vi "Esophogeal_HRME_Main_ImageCasting.vi"() -> ()   [LabVIEW 2021]
uses:
  typeDefs/Esophogeal_Software_States.ctl
  <vilib>/Utility/miscctls.llb/LVAllMonitorsDisplayTypeDef.ctl
  <vilib>/DAQmx/read.llb/DAQmx Read (Digital 1D Bool NChan 1Samp 1Line).vi
  <extravilib>/ChannelInstances/High Speed Stream-str/_Read For Replicate.vi
  <extravilib>/ChannelInstances/High Speed Stream-a[.,.](u8)/_Read For Replicate.vi
  <vilib>/DAQmx/create/channels.llb/DAQmx Create Channel (DI-Digital Input).vi
  <vilib>/DAQmx/miscellaneous.llb/DAQmx Fill In Error Info.vi
  <extravilib>/ChannelInstances/High Speed Stream-str/Instantiate.vi
  <extravilib>/ChannelInstances/High Speed Stream-a[.,.](u8)/Instantiate.vi
  <extravilib>/ChannelInstances/High Speed Stream-str/)Channel.vi
  <extravilib>/ChannelInstances/High Speed Stream-str/Abort Signal/Init Signal.vi
  <extravilib>/ChannelInstances/High Speed Stream-a[.,.](u8)/)Channel.vi
  <extravilib>/ChannelInstances/High Speed Stream-a[.,.](u8)/Abort Signal/Init Signal.vi
  <vilib>/vision/driver/NI_Vision_Acquisition_Software.lvlib
  <resource>/objmgr/imaqdx.rc
  <extravilib>/ChannelInstances/High Speed Stream-a[.,.](u8).lvlib
  <extravilib>/ChannelInstances/High Speed Stream-str.lvlib
  <vilib>/vision/NI_Vision_Development_Module.lvlib
panel:
  out "Pause Status":bool
  in  "Tab Control":enum32{"Main Page", "Image Session Info"}(tab)
  in  "MTN Threshold:":enum16{"24.0", "15.9"}(ring)
  in  "Calibrate":bool
  out "Image Analysis Meter":dbl(slide) scale=0.0..100.0
  out "Saved Imaged Number":i32=1 caption="Number of Images Saved"
  out "Image Save Notification":string
  in  "Auto Gain":bool=TRUE
  in  "Auto Exposure":bool=TRUE
  in  "Save Button":bool
  out "Recording":bool
  in  "Play Button":bool
  in  "Pause Button":bool
  in  "Close Program":bool
  in  "HRME Gain":dbl(slide)=18.0 scale=0.0..30.0
  in  "HRME Exposure":dbl(slide)=7000.0 scale=100.0..80000.0
  out "HRME Image":T1(plugin-control)
  out "Software States":T2
  out "HRME Path":path
  out "HRME Scores":path
  out "Representative Images":path
  out "error out":errorcluster
  out "Patient Folder":path
  in  "Command File Location":path=path "C:/Users/EsophaHRME_Dell3/Documents/GitHub/Esophageal_HRME_Software/EsophagealDeployment/Multi_Task_Network/CommandFiles/LabVIEW/cmds.json"
  out "Display:All Monitors":T3
  out "Width":i16
  out "Height":i16
  in  "Python Module Path":path=path "C:/Users/EsophaHRME_Dell3/Documents/GitHub/Esophageal_HRME_Software/EsophagealDeployment/Multi_Task_Network/mainv6.py"
  out "Log File Out":refnum<file>
  out "Timestamp":string
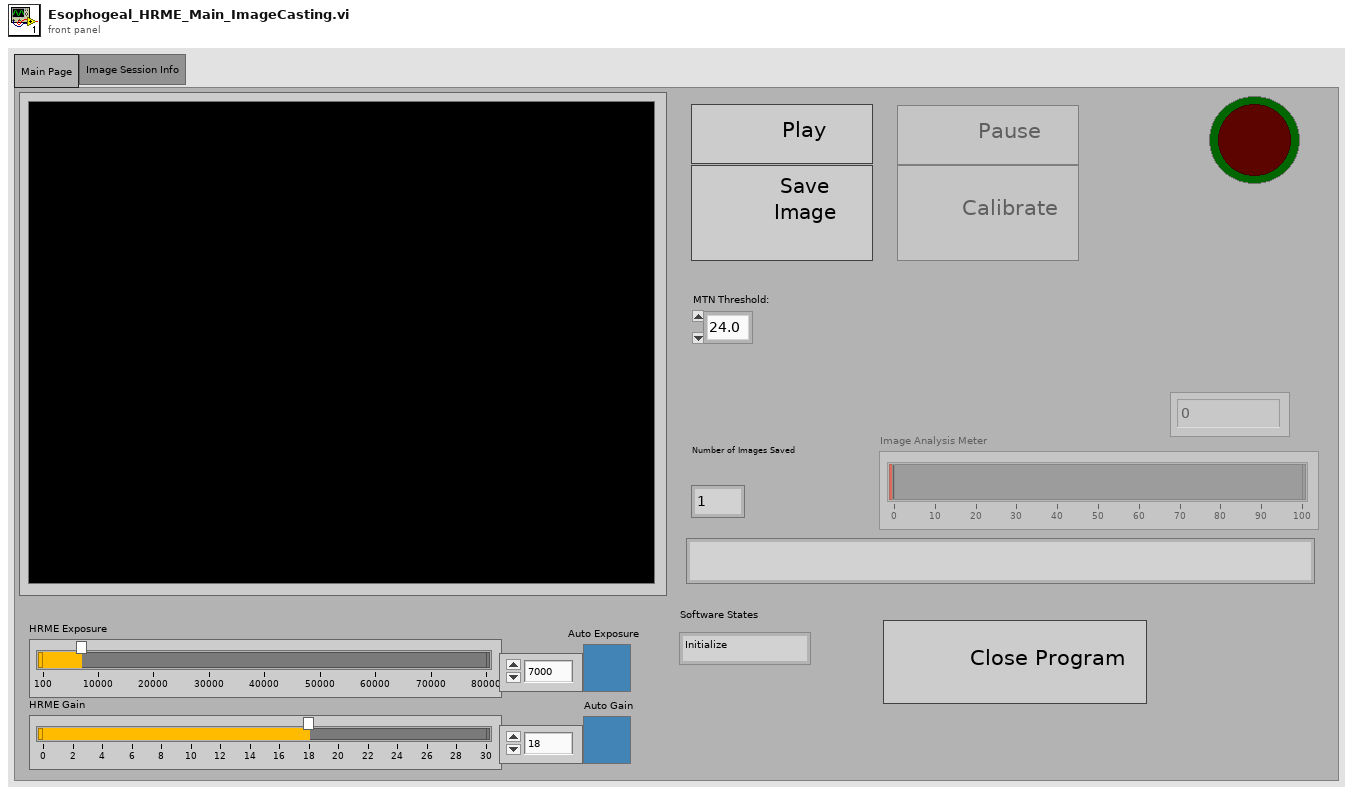
[diagram p1: front panel]
types:
  T1 = typedef "IMAQ Image.ctl" = refnum<image>
  T2 = typedef "Esophogeal_Software_States.ctl" = enum16{"Initialize", "Image Prep Screen", "Imaging", "Image Pause Screen", "Exit"}
  T3 = typedef "LVAllMonitorsDisplayTypeDef.ctl" = cluster{"Bounds":cluster{"Left":i16, "Top":i16, "Right":i16, "Bottom":i16}, "Depth":i16}[]
  T4 = enum8{"Enabled", "Disabled", "Disabled and Grayed Out"}
  T5 = enum16{"open", "replace", "create", "open or create", "replace or create", "replace or create with confirmation"}
  T6 = cluster{"Source":string, "Destination":string, "CMD":string, "Time":string}
  T7 = cluster{"Left":i32, "Top":i32, "Right":i32, "Bottom":i32}
  T8 = typedef "IMAQdx.ctl" = refnum<k21>
  T9 = cluster{"Bounds":cluster{"Left":i16, "Top":i16, "Right":i16, "Bottom":i16}, "Depth":i16}
  T10 = cluster{"Left":i16, "Top":i16, "Right":i16, "Bottom":i16}
  T11 = typedef "Image Type" = u32
  T12 = typedef "ROI Descriptor" = cluster{"Global Rectangle":i32[], "Contours":cluster{"ID":enum32{"External", "Internal"}, "Type":u32, "Coordinates":i32[]}[]}
  T13 = typedef "High Speed Stream-str.lvlib/)Channel.ctl" = refnum<queue>
  T14 = typedef "High Speed Stream-a[.,.](u8).lvlib/)Channel.ctl" = refnum<queue>
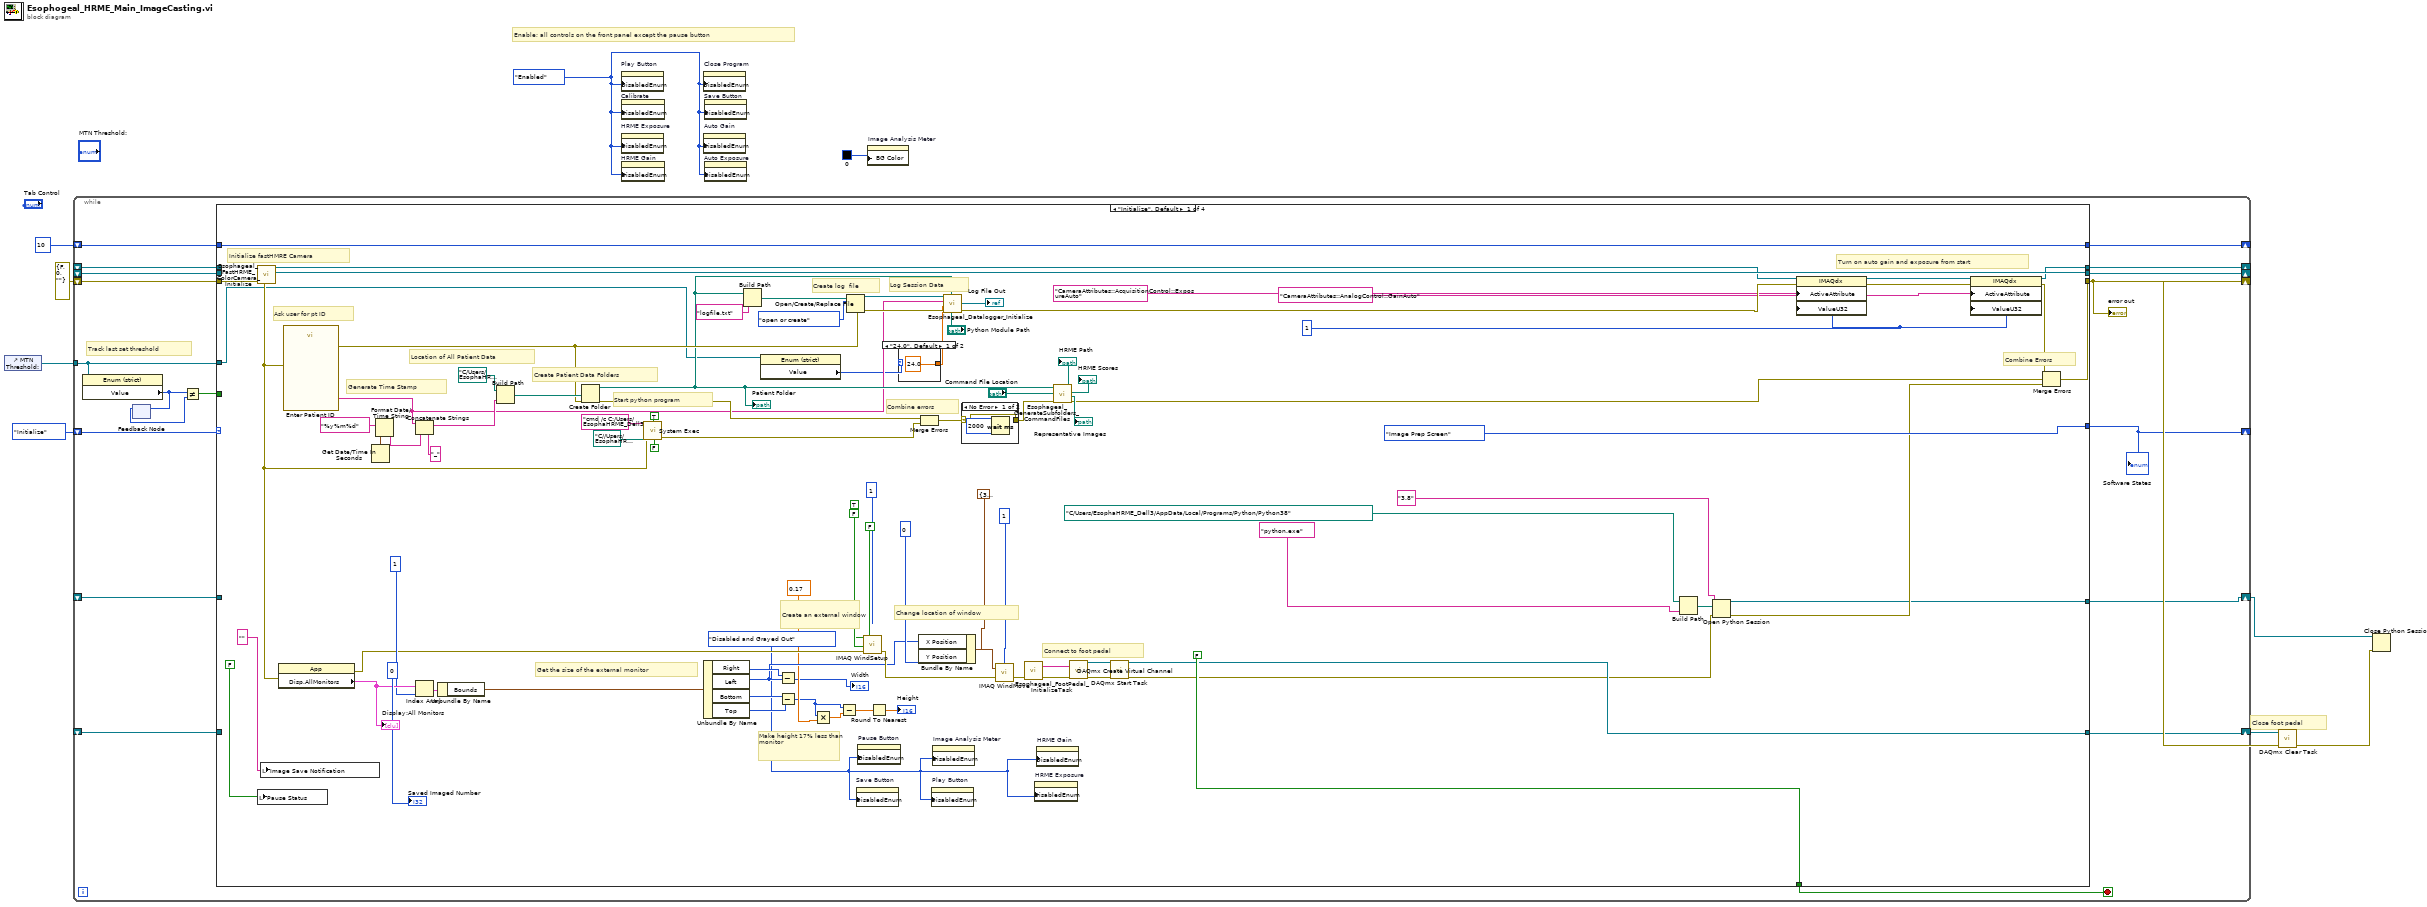
[diagram p0: block diagram]
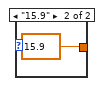
[diagram p2: hidden frame]
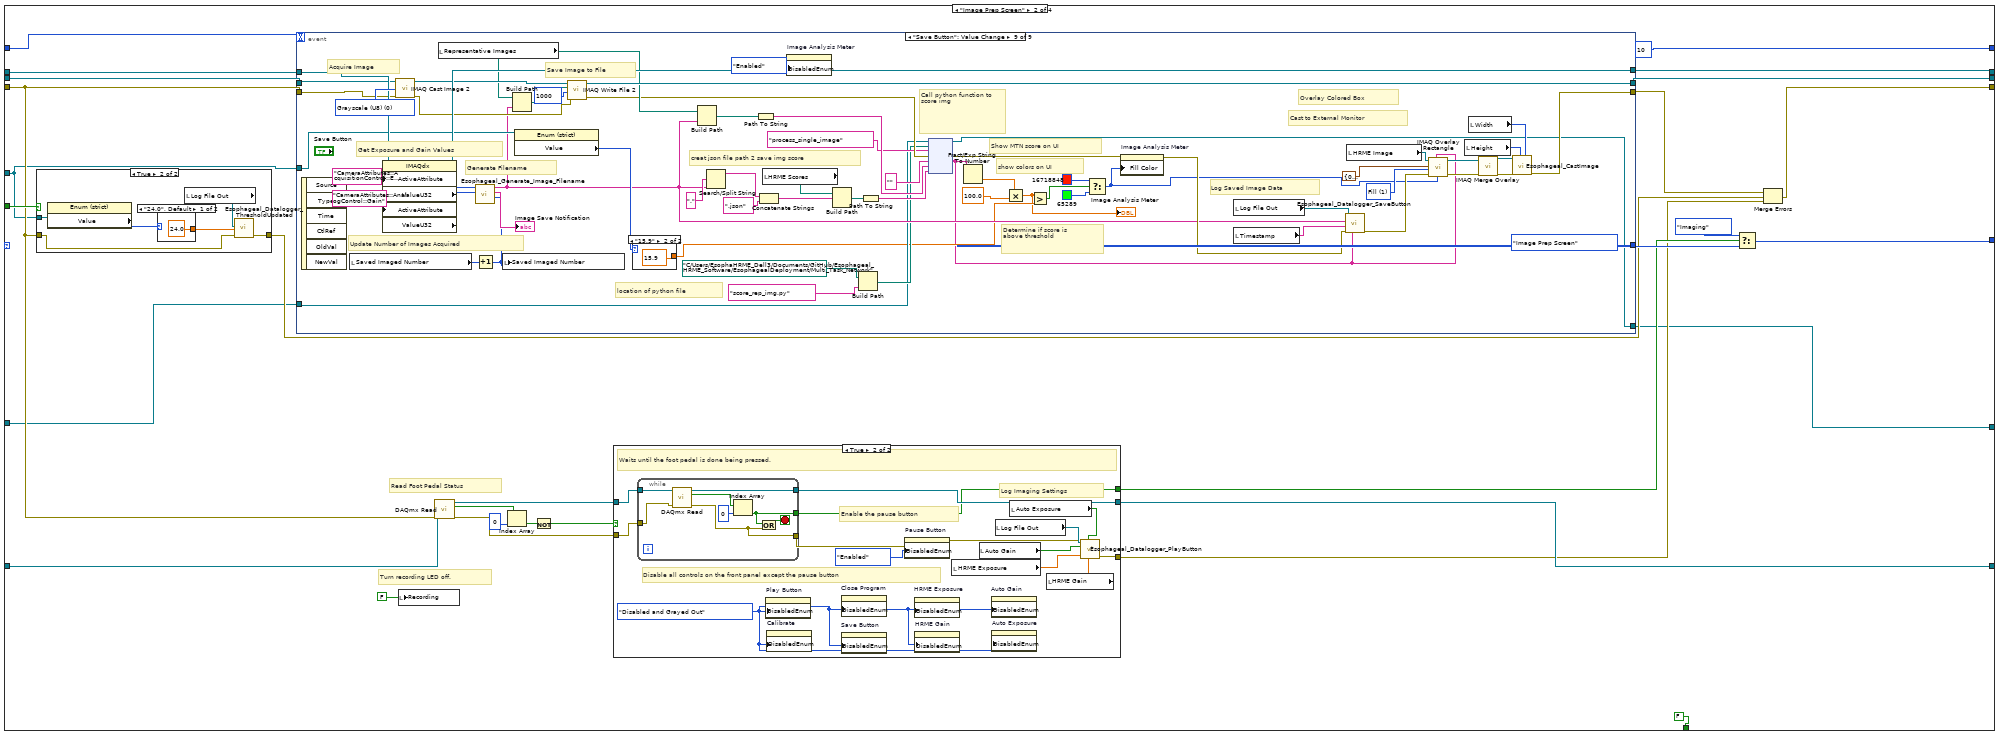
[diagram p4: hidden frame]
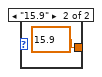
[diagram p6: hidden frame]
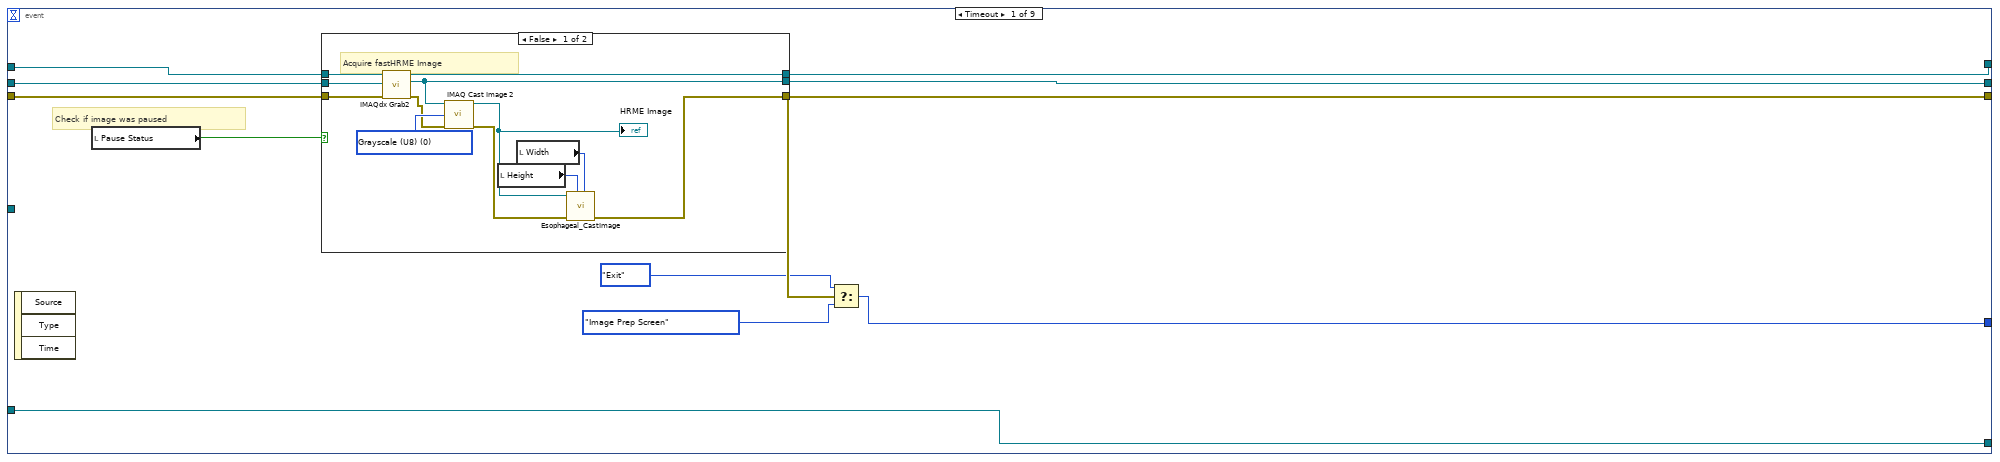
[diagram p8: hidden frame]
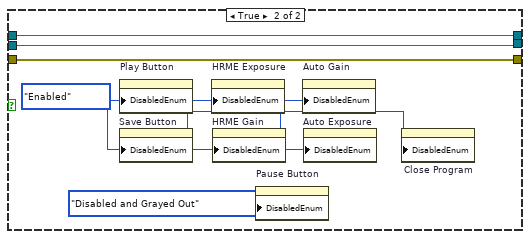
[diagram p9: hidden frame]
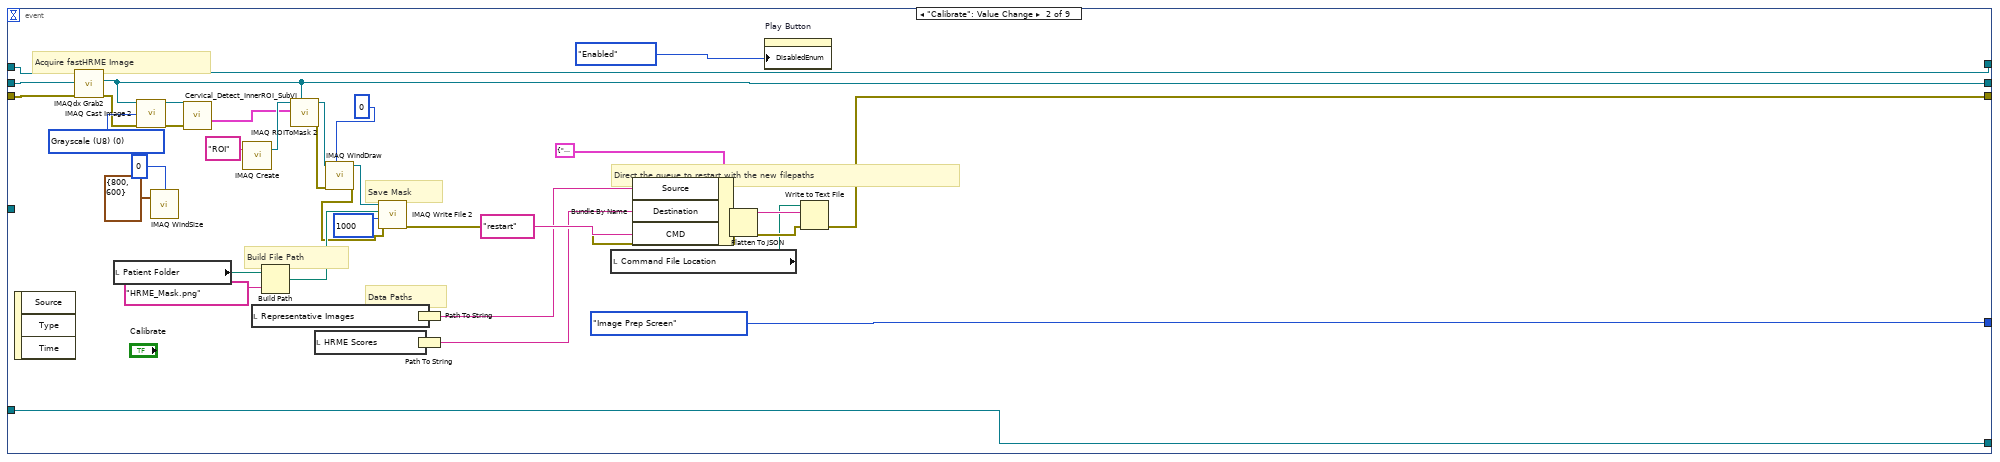
[diagram p10: hidden frame]
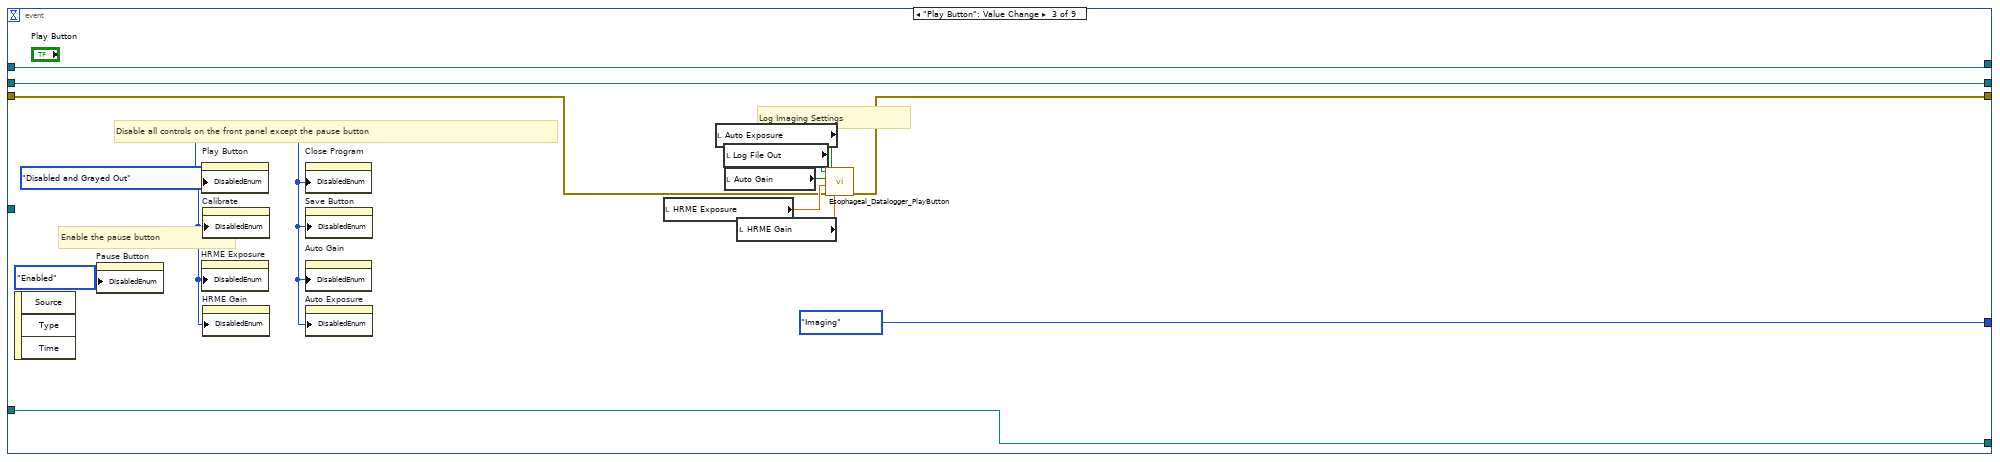
[diagram p11: hidden frame]
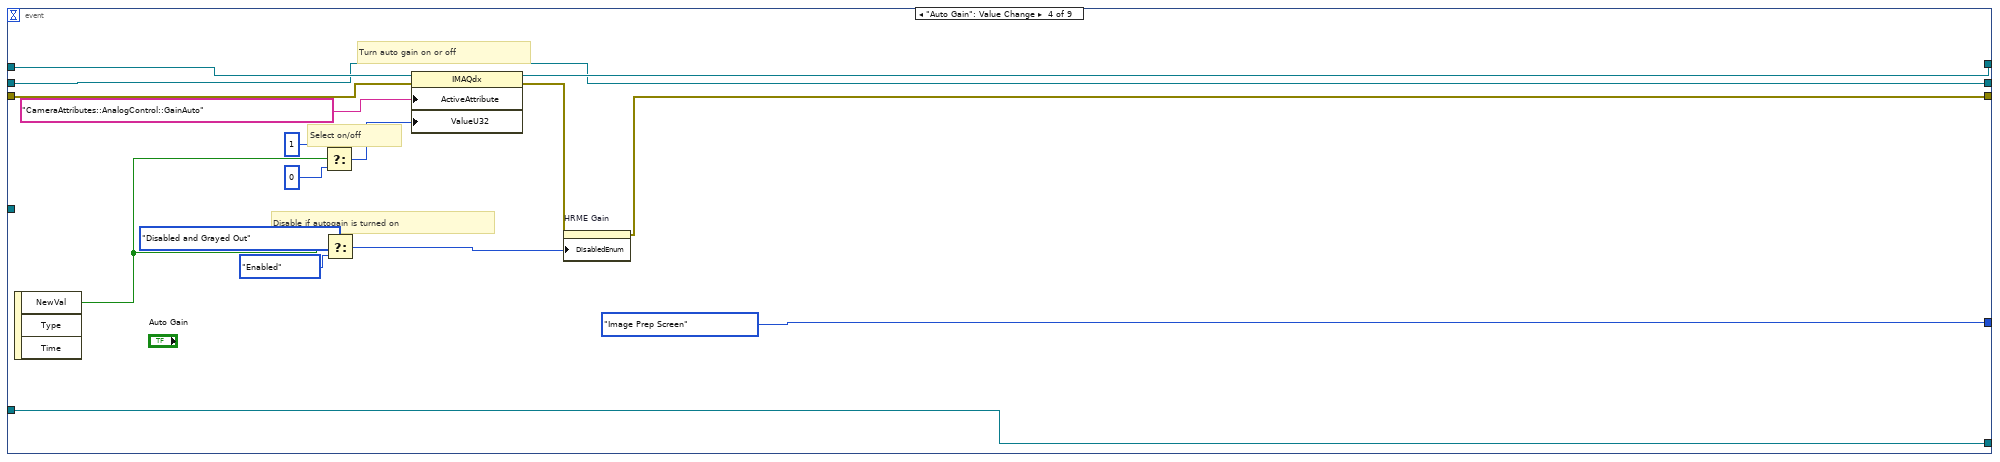
[diagram p12: hidden frame]
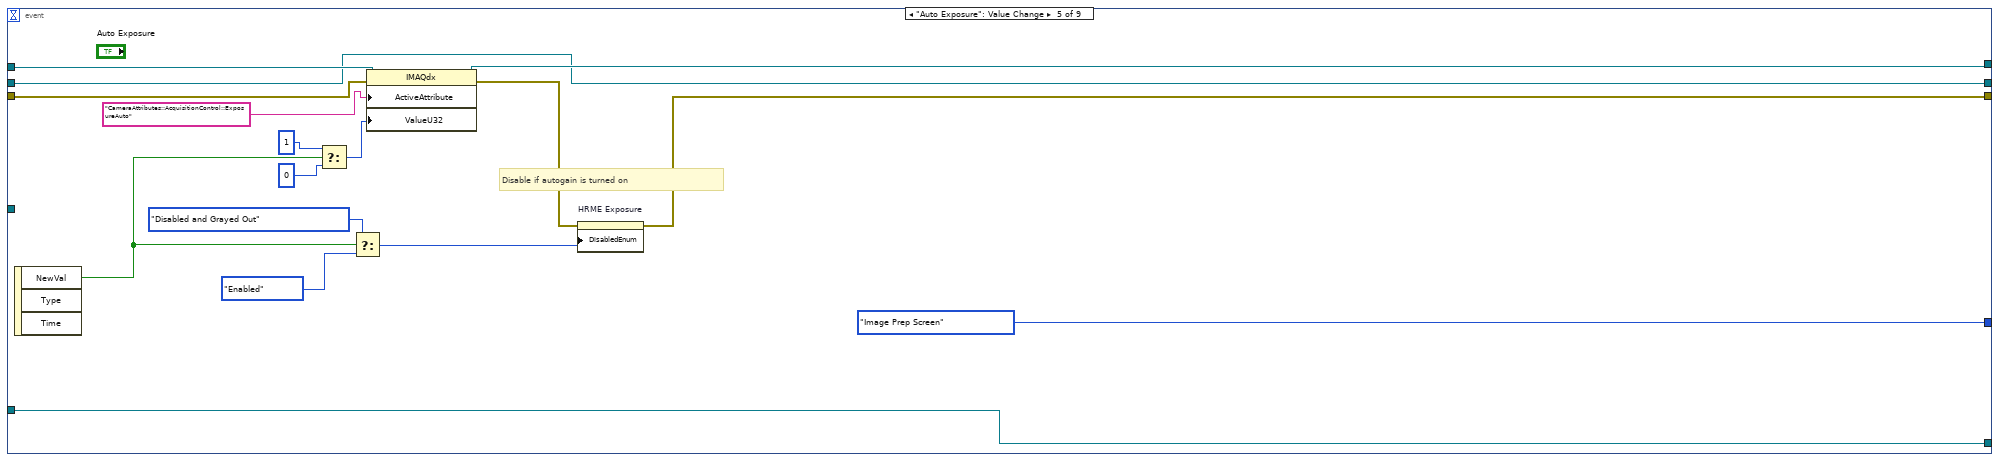
[diagram p13: hidden frame]
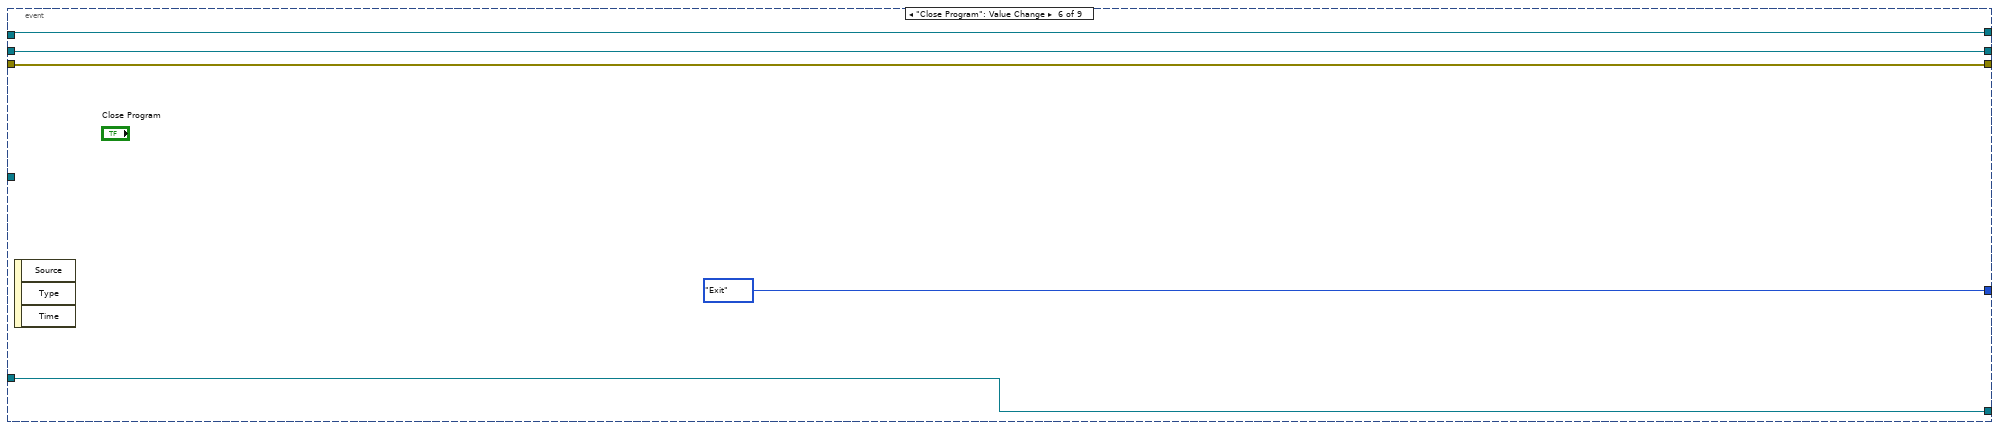
[diagram p14: hidden frame]
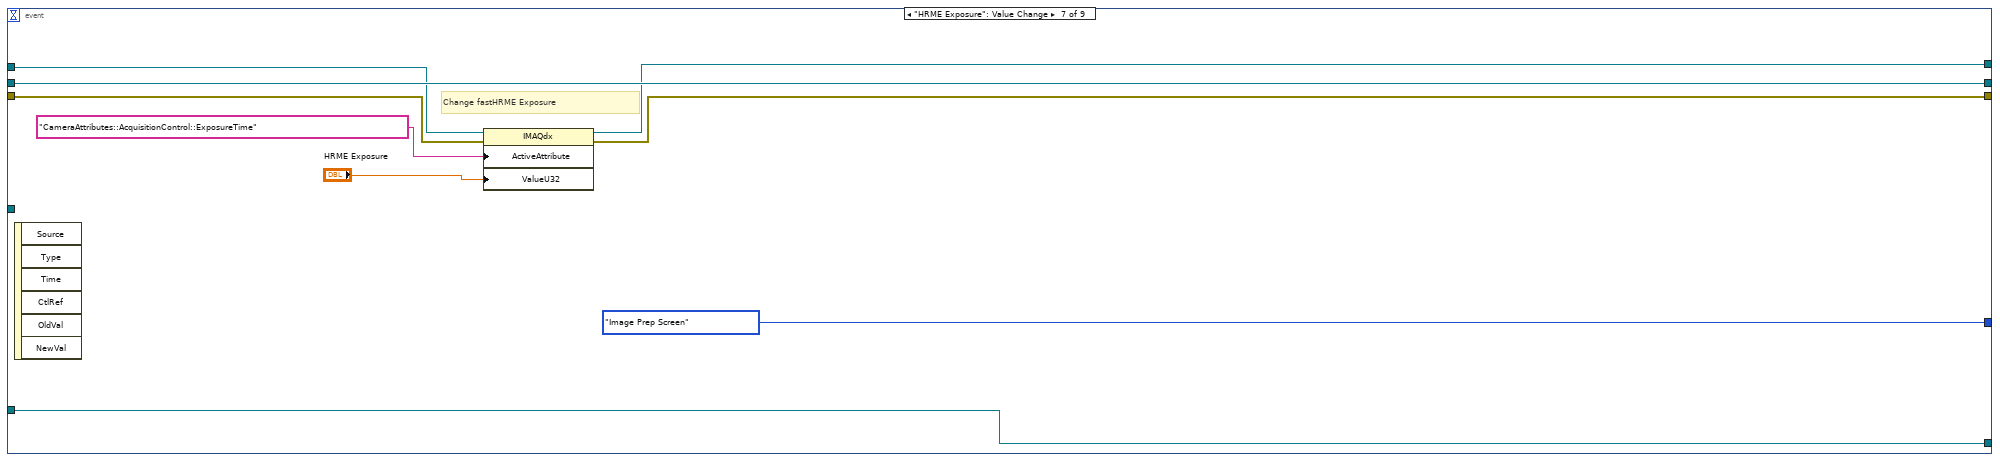
[diagram p15: hidden frame]
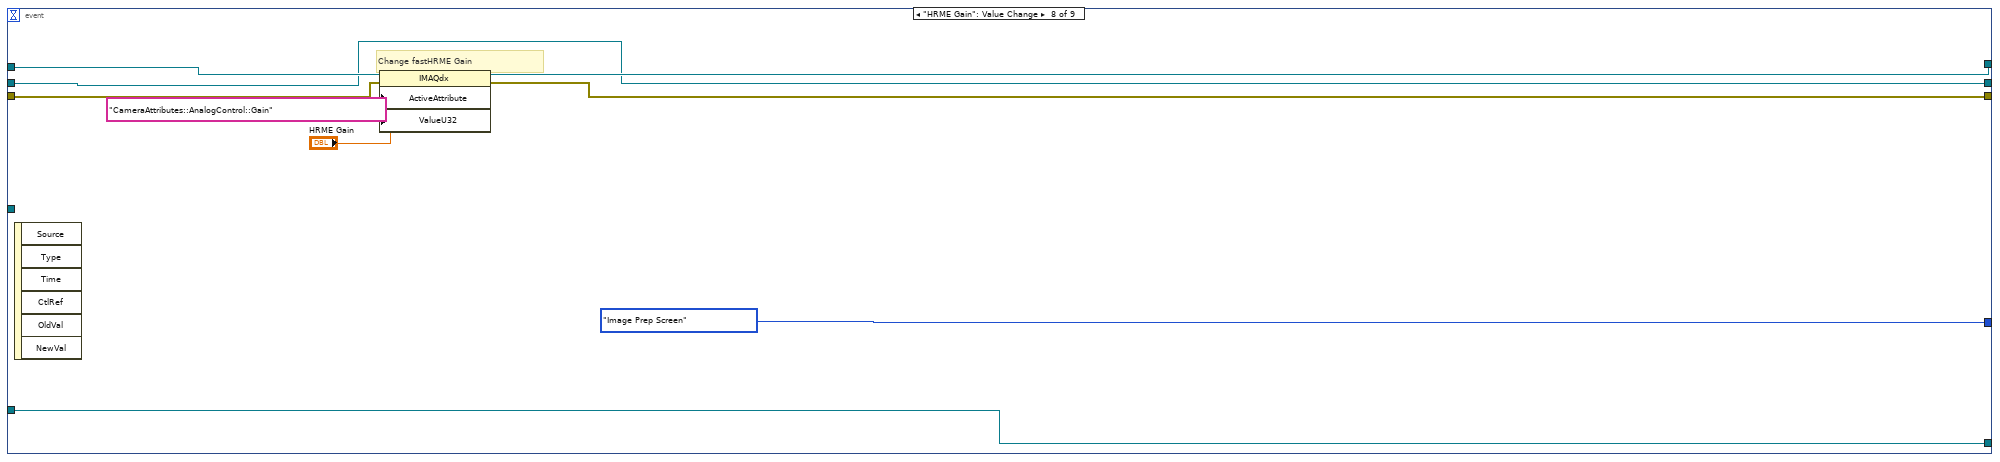
[diagram p16: hidden frame]
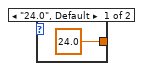
[diagram p17: hidden frame]
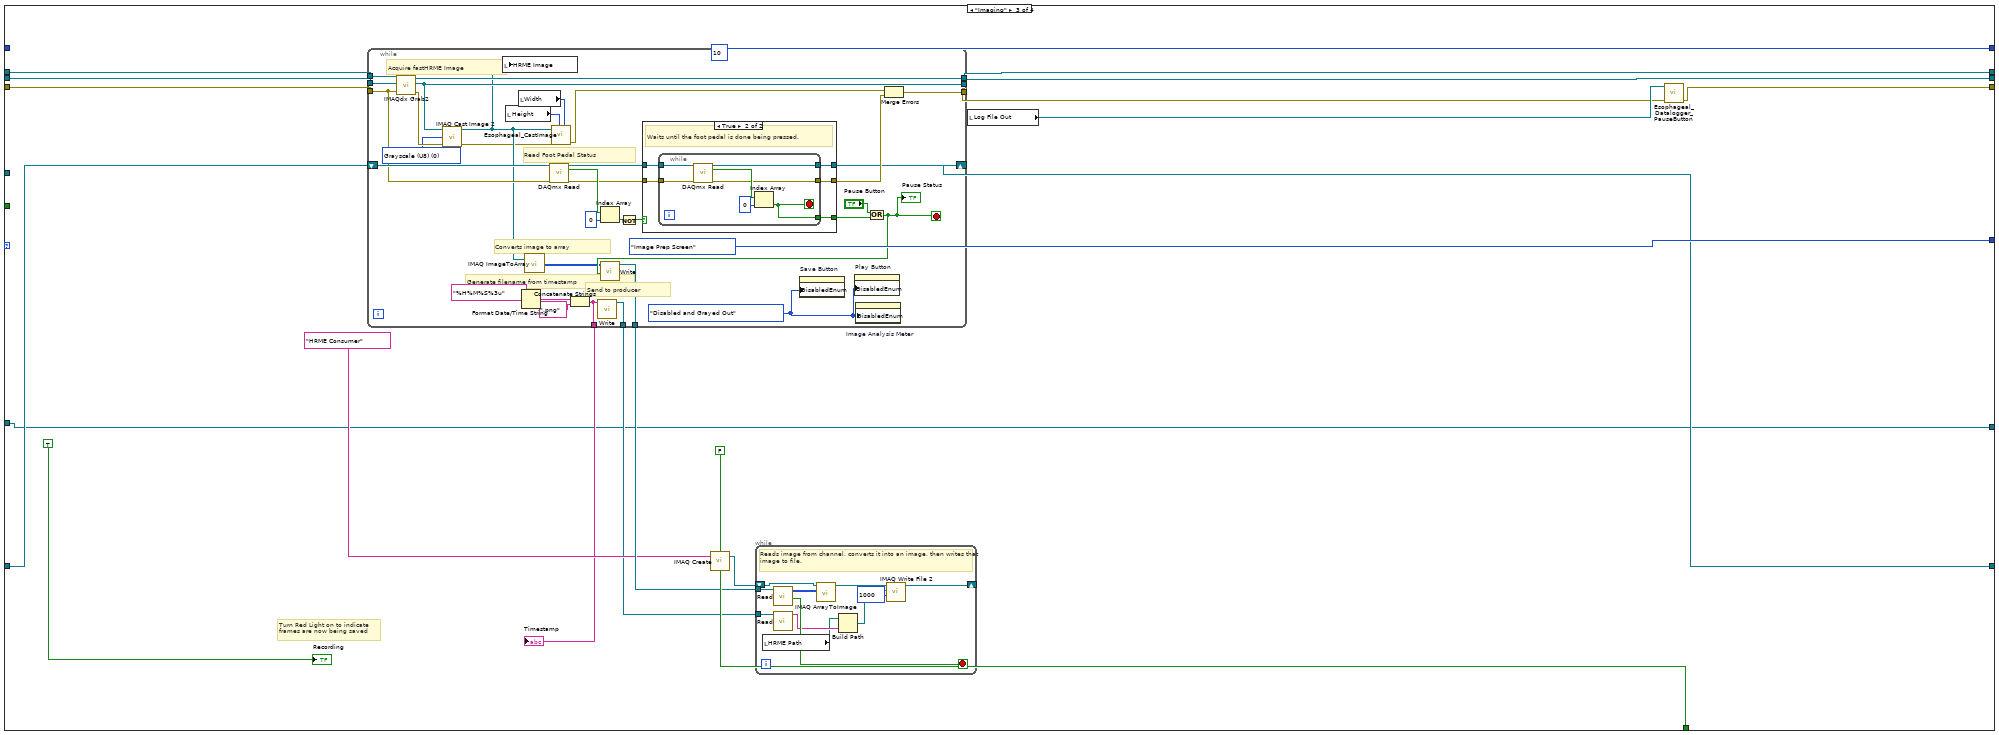
[diagram p18: hidden frame]
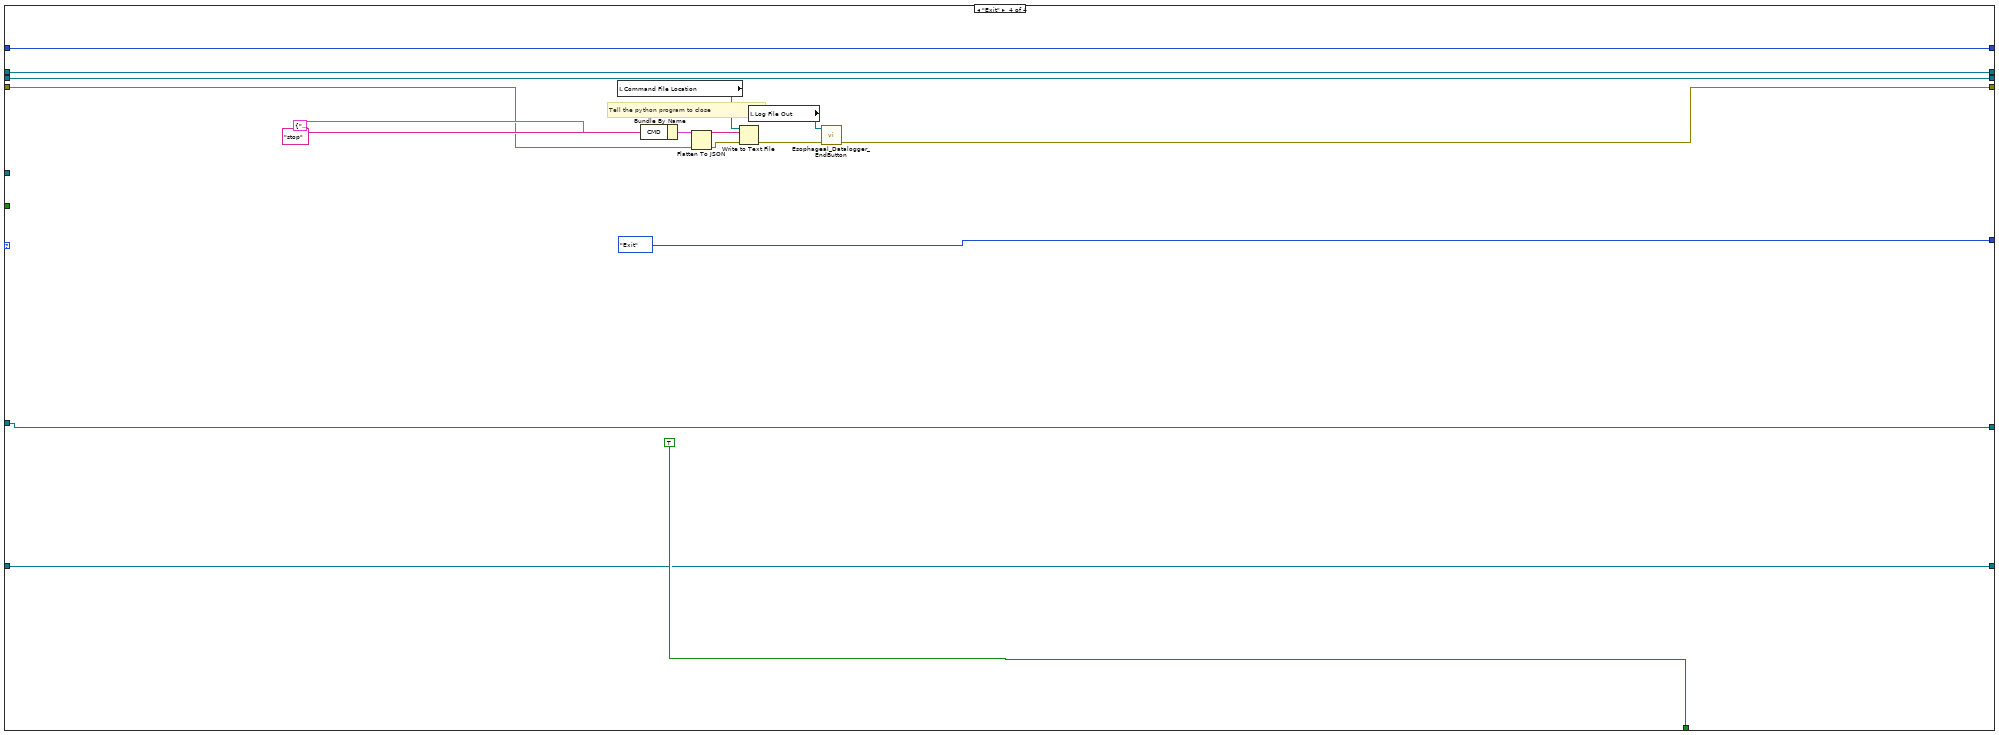
[diagram p20: hidden frame]
diagram:
  w5 = T4."Enabled" ("Disabled")
  # "Enable; all controls on the front panel except the pause button"
  # "Close foot pedal"
  n1 = control-ref of="MTN Threshold:"() -> (w3:refnum<vi>)
  n2 = while {
    shift-right: [w28] -> _
    shift-left: _ -> [w24]
    shift-right: [w27] -> _
    shift-left: _ -> [w23]
    shift-right: [w26] -> _
    shift-left: Esophogeal_Software_States."Initialize" ("Anal HRME States") -> [w29]
    shift-right: [w17] -> w8
    shift-left: errorcluster {"status"=FALSE, "code"=0, "source"=""} ("error IO") -> [w25]
    shift-right: [w20] -> w9
    shift-left: _ -> [w21]
    shift-right: [w18] -> _
    shift-left: 10 -> [w19]
    tunnel: w3 -> [w16]
    shift-right: [w12] -> w2
    shift-left: _ -> [w11]
    stop <- w22 stop-if-true
    # "Track last set threshold"
    n3 = property class="Enum (strict)"(reference=w16) -> ("Value"=w15:enum16{"24.0", "15.9"})  [unwired: 1 in, 2 out]
    n4 = feedback-in #1(w15) -> ()
    n5 = feedback #1() -> (w14:enum16{"24.0", "15.9"})  [unwired: 1 in]
    n6 = Not Equal?(x=w15, y=w14) -> (x != y?=w13:bool)
    n7 = case shown="\"Initialize\", Default" w29 {
      tunnel: [w38 w151 w403 w482] -> w28
      tunnel: [w119 w150 w402 w481] -> w27
      tunnel: [Esophogeal_Software_States."Image Prep Screen" ("Anal HRME States") w147 Esophogeal_Software_States."Image Prep Screen" ("Anal HRME States") Esophogeal_Software_States."Exit" ("Anal HRME States")] -> w26
      tunnel: w25 -> [w117 w130 w401 w471]
      tunnel: w24 -> [_ w153 w405 w482]
      tunnel: w23 -> [_ w152 w404 w481]
      tunnel: [FALSE FALSE FALSE TRUE] -> w22
      tunnel: [w103 w132 w392 w468] -> w17
      tunnel: w21 -> [_ w143 w400 w479]
      tunnel: [w113 w138 w397 w479] -> w20
      tunnel: w19 -> [w112 w136 _ w478]
      tunnel: [w112 10 10 w478] -> w18
      tunnel: w16 -> [w58 w127 _ _]
      tunnel: w13 -> [_ w131 _ _]
      tunnel: [w30 w125 w388 w467] -> w12
      tunnel: w11 -> [_ w126 w388 w467]
      frame "Initialize", Default {
        w40 = 1
        w37 = T4."Disabled and Grayed Out" ("Disabled")
        # "Combine errors"
        # "Turn on auto gain and exposure from start"
        # "Make height 17% less than monitor"
        # "Create log  file"
        # "Log Session Data"
        # "Change location of window"
        # "Create an external window"
        # "Get the size of the external monitor"
        # "Start python program"
        # "Location of All Patient Data"
        # "Combine Errors"
        # "Create Patient Data Folders"
        # "Generate Time Stamp"
        # "Ask user for pt ID"
        # "Connect to foot pedal"
        # "Initialize fastHMRE Camera"
        n8 = call "Esophageal_FastHRME_ColorCamera_Initialize.vi"("error in (no error)"=w117) -> ("error out"=w59:errorcluster, "HRME Image Reference"=w119:T1, "OMS Camera Reference Out"=w45:T8)  [unwired: 8 in]
        n9 = local write "Pause Status"(FALSE ("Pause Status")) -> ()
        n10 = local write "Image Save Notification"("" ("Image Save Notification")) -> ()
        n11 = property class="App"(error in=w59) -> (error out=w71:errorcluster, "Disp.AllMonitors"=w86:T3)  [unwired: 1 in, 1 out]
        "Display:All Monitors" <- w86
        n12 = call "Enter Patient ID"("error in (no error)"=w59) -> ("Patient ID"=w60:string, "error out"=w62:errorcluster)  [unwired: 16 in, 1 out]
        n13 = Get Date/Time In Seconds() -> (seconds since 1Jan1904=w109:timestamp)
        n14 = Format Date/Time String(time format string (%c)="%y%m%d", seconds (now)=w109) -> (date/time string=w106:string)  [unwired: 1 in]
        n15 = Concatenate Strings(w60, "_" ("string"), w106) -> (w105:string)
        n16 = Index Array(array=w86, index=1) -> (element=w84:T9)
        n17 = Unbundle By Name(w84) -> ("Bounds"=w83:T10)
        n18 = Build Path(base path=path "C:/Users/EsophaHRME_Dell3/Desktop/PatientData", name or relative path=w105) -> (appended path=w104:path)
        n19 = Create Folder(path (use dialog)=w104, error in=w62) -> (created path=w61:path, error out=w69:errorcluster)  [unwired: 1 in, 1 out]
        "Patient Folder" <- w61
        n20 = call <vilib>:"System Exec.vi"("run minimized? (F)"=TRUE, "wait until completion? (T)"=FALSE, "error in (no error)"=w59, "working directory"=path "C://Users/EsophaHRME_Dell3/Documents/GitHub/Esophageal_HRME_Software/EsophagealDeployment/Multi_Task_Network", "command line"="cmd /c C:/Users/EsophaHRME_Dell3/anaconda3/envs/esophaenv/python.exe \"C:/Users/EsophaHRME_Dell3/Documents/GitHub/Esophageal_HRME_Software/EsophagealDeployment/Multi_Task_Network/mainv6.py\"") -> ("error out"=w91:errorcluster)  [unwired: 3 in, 3 out]
        n21 = Unbundle By Name(w83) -> ("Right"=w82:i16, "Left"=w70:i16, "Bottom"=w81:i16, "Top"=w80:i16)
        n22 = Build Path(base path=w61, name or relative path="logfile.txt") -> (appended path=w68:path)
        n23 = property class="Enum (strict)"(reference=w58) -> ("Value"=w56:enum16{"24.0", "15.9"})  [unwired: 1 in, 2 out]
        n24 = Subtract(x=w82, y=w70) -> (x-y=→"Width":i16)
        n25 = Subtract(x=w81, y=w80) -> (x-y=w50:i16)
        n26 = Multiply(x=w50, y=0.17) -> (x*y=w51:dbl)
        n27 = Subtract(x=w50, y=w51) -> (x-y=w49:dbl)
        n28 = Open/Create/Replace File(file path (use dialog)=w68, error in=w62, operation (0:open)=T5."open or create") -> (refnum out=w66:refnum<file>, error out=w65:errorcluster)  [unwired: 3 in, 1 out]
        n29 = property on="Save Button" class="Bool"("DisabledEnum"=w37) -> ()  [unwired: 2 in, 2 out]
        n30 = property on="Pause Button" class="Bool"("DisabledEnum"=w37) -> ()  [unwired: 2 in, 2 out]
        n31 = call "IMAQ WindSetup"("Window is floating? (No)"=FALSE, "Window Number (0...15)"=1, "error in (no error)"=w71, "Window has title bar? (Yes)"=FALSE, "Window can grow? (Yes)"=TRUE ("Window has title bar? (Yes)")) -> ("error out"=w72:errorcluster)  [unwired: 6 in]
        n32 = Round To Nearest(number=w49) -> (nearest integer value=→"Height":dbl)
        n33 = case shown="\"24.0\", Default" w56 {
          tunnel: [24.0 15.9] -> w55
          frame "24.0", Default {
          }
          frame "15.9" {
          }
        }
        n34 = Bundle By Name(cluster=cluster{"X Position":i32, "Y Position":i32} {"X Position"=3840, "Y Position"=0} ("Coordinates (screen)"), "X Position"=w70, "Y Position"=0) -> (w76:cluster{"X Position":i32, "Y Position":i32})
        n35 = Merge Errors(w69, w91) -> (w92:errorcluster)
        n36 = property on="Play Button" class="Bool"("DisabledEnum"=w37) -> ()  [unwired: 2 in, 2 out]
        n37 = property on="Image Analysis Meter" class="Slide (strict)"("DisabledEnum"=w37) -> ()  [unwired: 2 in, 2 out]
        n38 = call "Esophageal_Datalogger_Initialize.vi"("Python Module Path"="Python Module Path", "Data File Path"=w61, "error in (no error)"=w65, "MTN Threshold"=w55, "Patient ID"=w60, "Log File In"=w66) -> ("error out"=w46:errorcluster, "Log File Out"=→"Log File Out":refnum<file>)  [unwired: 4 in]
        n39 = case shown="No Error" w92 {
          selector: w92 -> [w122 w124]
          tunnel: [w122 w124] -> w96
          frame No Error {
            n40 = Wait (ms)(milliseconds to wait=u32 2000) -> ()  [unwired: 1 out]
          }
          frame Error {
          }
        }
        n41 = call "IMAQ WindMove"("Window Number (0...15)"=1, "Coordinates (screen)"=w76, "error in (no error)"=w72) -> ("error out"=w73:errorcluster)  [unwired: 2 in, 1 out]
        n42 = call "Esophageal_FootPedal_InitializeTask.vi"("error in (no error)"=w73) -> ("error out"=w89:errorcluster, "Task Command"=w88:string)  [unwired: 9 in]
        n43 = property on="HRME Exposure" class="Slide (strict)"("DisabledEnum"=w37) -> ()  [unwired: 2 in, 2 out]
        n44 = property on="HRME Gain" class="Slide (strict)"("DisabledEnum"=w37) -> ()  [unwired: 2 in, 2 out]
        n45 = call "Esophageal_GenerateSubfolders_CommandFiles.vi"("error in"=w96, "Command File Location"="Command File Location", "Patient Data Folder"=w61) -> ("error out"=w97:errorcluster, "Rep Image Path"=→"Representative Images":path, "HRME Scores"=→"HRME Scores":path, "HRME Path"=→"HRME Path":path)  [unwired: 5 in]
        n46 = call-poly <vilib>:"DAQmx Create Virtual Channel.vi"("lines"=w88, "error in"=w89) -> ("task out"=w114:refnum<k21>, "error out"=w115:errorcluster)  [unwired: 12 in]
        n47 = call <vilib>:"DAQmx Start Task.vi"("task/channels in"=w114, "error in"=w115) -> ("task out"=w113:refnum<k21>, "error out"=w32:errorcluster)  [unwired: 12 in]
        n48 = Build Path(base path=path "C:/Users/EsophaHRME_Dell3/AppData/Local/Programs/Python/Python38", name or relative path="python.exe") -> (appended path=w35:path)
        n49 = Open Python Session(python version="3.8", python path=w35, 3:w32) -> (session out=w30:refnum<k35>, error out=w31:errorcluster)
        n50 = property class="IMAQdx"(reference=w45, error in=w46, "ActiveAttribute"="CameraAttributes::AcquisitionControl::ExposureAuto", "ValueU32"=w40) -> (reference out=w39:T8, error out=w42:errorcluster)
        n51 = property class="IMAQdx"(reference=w39, error in=w42, "ActiveAttribute"="CameraAttributes::AnalogControl::GainAuto", "ValueU32"=w40) -> (reference out=w38:T8, error out=w41:errorcluster)
        n52 = Merge Errors(w41, w97, w31) -> (w103:errorcluster)
        "Saved Imaged Number" <- 0
      }
      frame "Image Prep Screen" {
        # "Turn recording LED off."
        # "Read Foot Pedal Status"
        n53 = case shown="True" w131 {
          tunnel: w127 -> [_ w160]
          tunnel: w130 -> [w154 w156]
          tunnel: [w154 w155] -> w128
          frame False {
          }
          frame True {
            n54 = property class="Enum (strict)"(reference=w160) -> ("Value"=w159:enum16{"24.0", "15.9"})  [unwired: 1 in, 2 out]
            n55 = case shown="\"24.0\", Default" w159 {
              tunnel: [24.0 15.9] -> w158
              frame "24.0", Default {
              }
              frame "15.9" {
              }
            }
            n56 = local read "Log File Out"() -> (w157:refnum<file>)
            n57 = call "Esophageal_Datalogger_ThresholdUpdated.vi"("error in"=w156, "MTN Threshold"=w158, "Log File In"=w157) -> ("error out"=w155:errorcluster)  [unwired: 7 in, 1 out]
          }
        }
        n58 = event shown="[8] \"Save Button\": Value Change" {
          selector: _ -> [_ _ _ _ _ _ _ _ _]
          dyn-events: _ -> [_ _ _ _ _ _ _ _ _]
          timeout: w136 -> [_ _ _ _ _ _ _ _ _]
          tunnel: w153 -> [w198 w252 w265 w282 w295 w302 w310 w319 w369]
          tunnel: w152 -> [w196 w251 w264 w279 w292 w301 w311 w315 w368]
          tunnel: [w190 Esophogeal_Software_States."Image Prep Screen" ("Anal HRME States") Esophogeal_Software_States."Imaging" ("Anal HRME States") Esophogeal_Software_States."Image Prep Screen" ("Anal HRME States") Esophogeal_Software_States."Image Prep Screen" ("Anal HRME States") Esophogeal_Software_States."Exit" ("Anal HRME States") Esophogeal_Software_States."Image Prep Screen" ("Anal HRME States") Esophogeal_Software_States."Image Prep Screen" ("Anal HRME States") Esophogeal_Software_States."Image Prep Screen" ("Anal HRME States")] -> w146
          tunnel: [w197 w249 w265 w281 w294 w302 w309 w318 w380] -> w151
          tunnel: [w195 w227 w264 w279 w292 w301 w311 w315 w383] -> w150
          tunnel: w130 -> [w194 w250 w259 w280 w293 w300 w306 w316 w367]
          tunnel: [w191 w235 w258 w270 w288 w300 w305 w317 w364] -> w133
          tunnel: w127 -> [_ _ _ _ _ _ _ _ w352]
          tunnel: w126 -> [w188 w216 w254 w267 w283 w299 w304 w313 w332]
          tunnel: [w188 w216 w254 w267 w283 w299 w304 w313 w325] -> w125
          event Timeout {
            # "Check if image was paused"
            n59 = event-data() -> ()  [unwired: 1 in, 3 out]
            n60 = local read "Pause Status"() -> (w193:bool)
            n61 = case shown="False" w193 {
              tunnel: w198 -> [w210 w215]
              tunnel: [w209 w215] -> w197
              tunnel: w196 -> [w208 w214]
              tunnel: [w206 w214] -> w195
              tunnel: w194 -> [w207 w212]
              tunnel: [w201 w212] -> w191
              frame False {
                w205 = T11 0 items=["Grayscale (U8)", "Grayscale (I16)", "Grayscale (SGL)", "Complex (CSG)", "RGB (U32)", "HSL (U32)", "RGB (U64)", "Grayscale (U16)"] ("Image Type")
                # "Acquire fastHRME Image"
                n62 = call <vilib>:"IMAQdx Grab2.vi"("error in"=w207, "Image In"=w208, "Session In"=w210) -> ("error out"=w203:errorcluster, "Image Out"=w206:T1, "Session Out"=w209:T8)  [unwired: 5 in, 1 out]
                n63 = call "IMAQ Cast Image 2"("Image Src"=w206, "Image Type"=w205, "error in (no error)"=w203) -> ("Image Dst Out"=w204:T1, "error out"=w202:errorcluster)  [unwired: 11 in]
                "HRME Image" <- w204
                n64 = local read "Height"() -> (w200:i16)
                n65 = local read "Width"() -> (w199:i16)
                n66 = call "Esophageal_CastImage.vi"("X Resolution"=w199, "Y Resolution"=w200, "error in (no error)"=w202, "Image In"=w204) -> ("error out"=w201:errorcluster)  [unwired: 7 in]
              }
              frame True {
                w211 = T4."Enabled" ("Disabled")
                n67 = property on="Play Button" class="Bool"("DisabledEnum"=w211) -> ()  [unwired: 2 in, 2 out]
                n68 = property on="Save Button" class="Bool"("DisabledEnum"=w211) -> ()  [unwired: 2 in, 2 out]
                n69 = property on="HRME Exposure" class="Slide (strict)"("DisabledEnum"=w211) -> ()  [unwired: 2 in, 2 out]
                n70 = property on="HRME Gain" class="Slide (strict)"("DisabledEnum"=w211) -> ()  [unwired: 2 in, 2 out]
                n71 = property on="Pause Button" class="Bool"("DisabledEnum"=T4."Disabled and Grayed Out" ("Disabled")) -> ()  [unwired: 2 in, 2 out]
                n72 = property on="Auto Gain" class="Bool (strict)"("DisabledEnum"=w211) -> ()  [unwired: 2 in, 2 out]
                n73 = property on="Auto Exposure" class="Bool (strict)"("DisabledEnum"=w211) -> ()  [unwired: 2 in, 2 out]
                n74 = property on="Close Program" class="Bool"("DisabledEnum"=w211) -> ()  [unwired: 2 in, 2 out]
              }
            }
            n75 = Select(t=Esophogeal_Software_States."Exit" ("Anal HRME States"), s=w191, f=Esophogeal_Software_States."Image Prep Screen" ("Anal HRME States")) -> (s? t:f=w190:T2)
          }
          event "Calibrate": Value Change {
            w253 = T11 0 items=["Grayscale (U8)", "Grayscale (I16)", "Grayscale (SGL)", "Complex (CSG)", "RGB (U32)", "HSL (U32)", "RGB (U64)", "Grayscale (U16)"] ("Image Type")
            # "Data Paths"
            # "Direct the queue to restart with the new filepaths"
            # "Build File Path"
            # "Save Mask"
            # "Acquire fastHRME Image"
            n76 = event-data() -> ()  [unwired: 1 in, 3 out]
            n77 = call <vilib>:"IMAQdx Grab2.vi"("error in"=w250, "Image In"=w251, "Session In"=w252) -> ("error out"=w241:errorcluster, "Image Out"=w227:T1, "Session Out"=w249:T8)  [unwired: 5 in, 1 out]
            n78 = local read "Patient Folder"() -> (w247:path)
            n79 = call "IMAQ Cast Image 2"("Image Src"=w227, "Image Type"=w253, "error in (no error)"=w241) -> ("Image Dst Out"=w223:T1, "error out"=w222:errorcluster)  [unwired: 11 in]
            n80 = call "IMAQ WindSize"("Width & Height"=cluster{"Width":i32, "Height":i32} {"Width"=800, "Height"=600}, "Window Number"=0) -> ()  [unwired: 4 in, 3 out]
            n81 = call "Cervical_Detect_InnerROI_SubVI.vi"("error in"=w222, "Raw Image"=w223) -> ("ROI Descriptor"=w221:T12)  [unwired: 6 in, 3 out]
            n82 = call "IMAQ Create"("Image Name"="ROI") -> ("New Image"=w242:T1)  [unwired: 4 in, 1 out]
            n83 = local read "Representative Images"() -> (w232:path)
            n84 = Build Path(base path=w247, name or relative path="HRME_Mask.png") -> (appended path=w245:path)
            n85 = call "IMAQ ROIToMask 2"("Image Model"=w227, "ROI Descriptor"=w221, "Image"=w242) -> ("error out"=w219:errorcluster, "Image Out"=w220:T1)  [unwired: 6 in, 1 out]
            n86 = local read "HRME Scores"() -> (w231:path)
            n87 = call "IMAQ WindDraw"("Window Number (0...15)"=0 ("Window Number (-1...15)"), "error in (no error)"=w219, "Image"=w220) -> ("error out"=w217:errorcluster, "Image Out (duplicate)"=w218:T1)  [unwired: 7 in]
            n88 = call-poly "IMAQ Write File 2"("error in (no error)"=w217, "Image Quality"=u32 1000, "File Path"=w245, "Image"=w218) -> ("error out"=w237:errorcluster)  [unwired: 6 in, 1 out]
            n89 = Path To String(path=w232) -> (string=w230:string)
            n90 = Path To String(path=w231) -> (string=w229:string)
            n91 = local read "Command File Location"() -> (w233:path)
            n92 = Bundle By Name(cluster=T6 {"Source"="", "Destination"="", "CMD"="newfolders", "Time"="time"} ("Output JSON File"), "Source"=w230, "Destination"=w229, "CMD"="restart") -> (w239:T6)
            n93 = Flatten To JSON(anything=w239, error in (no error)=w237) -> (JSON string=w240:string, 11:w236:errorcluster)  [unwired: 1 in]
            n94 = property on="Play Button" class="Bool"("DisabledEnum"=T4."Enabled" ("Disabled")) -> ()  [unwired: 2 in, 2 out]
            n95 = Write to Text File(file (use dialog)=w233, text=w240, error in=w236) -> (error out=w235:errorcluster)  [unwired: 1 in, 2 out]
          }
          event "Play Button": Value Change {
            w262 = T4."Disabled and Grayed Out" ("Disabled")
            # "Log Imaging Settings"
            # "Enable the pause button"
            # "Disable all controls on the front panel except the pause button"
            n96 = event-data() -> ()  [unwired: 1 in, 3 out]
            n97 = property on="Pause Button" class="Bool"("DisabledEnum"=T4."Enabled" ("Disabled")) -> ()  [unwired: 2 in, 2 out]
            n98 = property on="Play Button" class="Bool"("DisabledEnum"=w262) -> ()  [unwired: 2 in, 2 out]
            n99 = property on="HRME Exposure" class="Slide (strict)"("DisabledEnum"=w262) -> ()  [unwired: 2 in, 2 out]
            n100 = property on="Calibrate" class="Bool"("DisabledEnum"=w262) -> ()  [unwired: 2 in, 2 out]
            n101 = property on="HRME Gain" class="Slide (strict)"("DisabledEnum"=w262) -> ()  [unwired: 2 in, 2 out]
            n102 = property on="Close Program" class="Bool"("DisabledEnum"=w262) -> ()  [unwired: 2 in, 2 out]
            n103 = property on="Auto Gain" class="Bool (strict)"("DisabledEnum"=w262) -> ()  [unwired: 2 in, 2 out]
            n104 = property on="Save Button" class="Bool"("DisabledEnum"=w262) -> ()  [unwired: 2 in, 2 out]
            n105 = property on="Auto Exposure" class="Bool (strict)"("DisabledEnum"=w262) -> ()  [unwired: 2 in, 2 out]
            n106 = local read "HRME Exposure"() -> (w260:dbl)
            n107 = local read "Auto Exposure"() -> (w257:bool)
            n108 = local read "Log File Out"() -> (w255:refnum<file>)
            n109 = local read "Auto Gain"() -> (w256:bool)
            n110 = local read "HRME Gain"() -> (w261:dbl)
            n111 = call "Esophageal_Datalogger_PlayButton.vi"("Gain Value"=w261, "Auto Exposure Status"=w257, "error in (no error)"=w259, "Exposure Value"=w260, "Auto Gain Status"=w256, "Log File In"=w255) -> ("error out"=w258:errorcluster)  [unwired: 4 in, 1 out]
          }
          event "Auto Gain": Value Change {
            # "Disable if autogain is turned on"
            # "Select on/off"
            # "Turn auto gain on or off"
            n112 = event-data() -> ("NewVal"=w273:bool)  [unwired: 1 in, 2 out]
            n113 = Select(t=u32 1 ("ValueU32"), s=w273, f=u32 0 ("ValueU32")) -> (s? t:f=w276:u32)
            n114 = Select(t=T4."Disabled and Grayed Out" ("Disabled"), s=w273, f=T4."Enabled" ("Disabled")) -> (s? t:f=w272:T4)
            n115 = property class="IMAQdx"(reference=w282, error in=w280, "ActiveAttribute"="CameraAttributes::AnalogControl::GainAuto", "ValueU32"=w276) -> (reference out=w281:T8, error out=w271:errorcluster)
            n116 = property on="HRME Gain" class="Slide (strict)"(error in=w271, "DisabledEnum"=w272) -> (error out=w270:errorcluster)  [unwired: 1 in, 1 out]
          }
          event "Auto Exposure": Value Change {
            # "Disable if autogain is turned on"
            n117 = event-data() -> ("NewVal"=w286:bool)  [unwired: 1 in, 2 out]
            n118 = Select(t=u32 1 ("ValueU32"), s=w286, f=u32 0 ("ValueU32")) -> (s? t:f=w298:u32)
            n119 = Select(t=T4."Disabled and Grayed Out" ("Disabled"), s=w286, f=T4."Enabled" ("Disabled")) -> (s? t:f=w287:T4)
            n120 = property class="IMAQdx"(reference=w295, error in=w293, "ActiveAttribute"="CameraAttributes::AcquisitionControl::ExposureAuto", "ValueU32"=w298) -> (reference out=w294:T8, error out=w289:errorcluster)
            n121 = property on="HRME Exposure" class="Slide (strict)"(error in=w289, "DisabledEnum"=w287) -> (error out=w288:errorcluster)  [unwired: 1 in, 1 out]
          }
          event "Close Program": Value Change {
            n122 = event-data() -> ()  [unwired: 1 in, 3 out]
          }
          event "HRME Exposure": Value Change {
            # "Change fastHRME Exposure"
            n123 = event-data() -> ()  [unwired: 1 in, 6 out]
            n124 = property class="IMAQdx"(reference=w310, error in=w306, "ActiveAttribute"="CameraAttributes::AcquisitionControl::ExposureTime", "ValueU32"="HRME Exposure") -> (reference out=w309:T8, error out=w305:errorcluster)
          }
          event "HRME Gain": Value Change {
            # "Change fastHRME Gain"
            n125 = event-data() -> ()  [unwired: 1 in, 6 out]
            n126 = property class="IMAQdx"(reference=w319, error in=w316, "ActiveAttribute"="CameraAttributes::AnalogControl::Gain", "ValueU32"="HRME Gain") -> (reference out=w318:T8, error out=w317:errorcluster)
          }
          event "Save Button": Value Change {
            w357 = u32 1 items=["Frame", "Fill", "Highlight"] ("Drawing Mode (Frame)")
            w373 = T11 0 items=["Grayscale (U8)", "Grayscale (I16)", "Grayscale (SGL)", "Complex (CSG)", "RGB (U32)", "HSL (U32)", "RGB (U64)", "Grayscale (U16)"] ("Image Type")
            # "creat json file path 2 save img score"
            # "Determine if score is \nabove threshold"
            # "Show MTN score on UI"
            # "show colors on UI"
            # "Call python function to score img"
            # "location of python file"
            # "Log Saved Image Data"
            # "Overlay Colored Box"
            # "Cast to External Monitor"
            # "Update Number of Images Acquired"
            # "Generate Filename"
            # "Acquire Image"
            # "Get Exposure and Gain Values"
            # "Save Image to File"
            n127 = event-data() -> ()  [unwired: 1 in, 6 out]
            n128 = local read "Saved Imaged Number"() -> (w376:i32)
            n129 = property class="IMAQdx"(reference=w369, "ActiveAttribute"="CameraAttributes::AcquisitionControl::ExposureTime", "ActiveAttribute"="CameraAttributes::AnalogControl::Gain") -> (reference out=w380:T8, "ValueU32"=w379:u32, "ValueU32"=w378:u32)  [unwired: 1 in, 1 out]
            n130 = call "IMAQ Cast Image 2"("Image Src"=w368, "Image Type"=w373, "error in (no error)"=w367) -> ("Image Dst Out"=w372:T1, "error out"=w371:errorcluster)  [unwired: 11 in]
            n131 = local read "Representative Images"() -> (w348:path)
            n132 = Increment(x=w376) -> (x+1=w374:i32)
            n133 = call "Esophageal_Generate_Image_Filename.vi"("Image Number"=w374, "HRME Gain"=w378, "HRME Exposure"=w379) -> ("Notification Text"=→"Image Save Notification":string, "Image Filename"=w342:string)  [unwired: 7 in]
            n134 = local write "Saved Imaged Number"(w374) -> ()
            n135 = Build Path(base path=w348, name or relative path=w342) -> (appended path=w385:path)
            n136 = property class="Enum (strict)"(reference=w352) -> ("Value"=w351:enum16{"24.0", "15.9"})  [unwired: 1 in, 2 out]
            n137 = call-poly "IMAQ Write File 2"("error in (no error)"=w371, "Image Quality"=u32 1000, "File Path"=w385, "Image"=w372) -> ("error out"=w336:errorcluster, "Image Out (duplicate)"=w383:T1)  [unwired: 6 in]
            n138 = case shown="\"15.9\"" w351 {
              tunnel: [24.0 15.9] -> w326
              frame "24.0", Default {
              }
              frame "15.9" {
              }
            }
            n139 = Build Path(base path=w348, name or relative path=w342) -> (appended path=w340:path)
            n140 = Search/Split String(string=w342, search string/char (-)=".") -> (substring before match=w345:string)  [unwired: 1 in, 2 out]
            n141 = Path To String(path=w340) -> (string=w339:string)
            n142 = Concatenate Strings(w345, ".json") -> (w344:string)
            n143 = local read "HRME Scores"() -> (w341:path)
            n144 = property on="Image Analysis Meter" class="Slide (strict)"("DisabledEnum"=T4."Enabled" ("Disabled")) -> ()  [unwired: 2 in, 2 out]
            n145 = Build Path(base path=w341, name or relative path=w344) -> (appended path=w343:path)
            n146 = Build Path(base path=path "C:/Users/EsophaHRME_Dell3/Documents/GitHub/Esophageal_HRME_Software/EsophagealDeployment/Multi_Task_Network", name or relative path="score_rep_img.py") -> (appended path=w333:path)
            n147 = Path To String(path=w343) -> (string=w338:string)
            n148 = node(w332, w333, "process_single_image", w336, "", w339, w338) -> (w325:refnum<k35>, w335:errorcluster, w323:string)  [unwired: 2 in, 2 out]
            n149 = Fract/Exp String To Number(string=w323) -> (number=w327:dbl)  [unwired: 3 in, 1 out]
            n150 = Multiply(x=w327, y=100.0) -> (x*y=w324:dbl)
            "Image Analysis Meter" <- w324
            n151 = Greater?(x=w324, y=w326) -> (0:w331:bool)
            n152 = Select(t=u32 16718848, s=w331, f=u32 65289) -> (s? t:f=w322:u32)
            n153 = property on="Image Analysis Meter" class="Slide (strict)"(error in=w335, "Fill Color"=w322) -> (error out=w354:errorcluster)  [unwired: 1 in, 1 out]
            n154 = local read "Log File Out"() -> (w356:refnum<file>)
            n155 = local read "Timestamp"() -> (w355:string)
            n156 = call "Esophageal_Datalogger_SaveButton.vi"("HRME Score"=w323, "error in (no error)"=w354, "Timestamp"=w355, "Image Name"=w342, "Log File In"=w356) -> ("error out"=w353:errorcluster)  [unwired: 5 in, 1 out]
            n157 = local read "HRME Image"() -> (w363:T1)
            n158 = call "IMAQ Overlay Rectangle"("Color"=w322, "Group"=w323, "error in (no error)"=w353, "Drawing Mode (Frame)"=w357, "Rectangle"=T7 {"Left"=0, "Top"=0, "Right"=50, "Bottom"=50}, "Image"=w363) -> ("error out"=w359:errorcluster, "Image Out"=w362:T1)  [unwired: 4 in]
            n159 = local read "Height"() -> (w366:i16)
            n160 = local read "Width"() -> (w365:i16)
            n161 = call "IMAQ Merge Overlay"("error in (no error)"=w359, "Image Src"=w362) -> ("error out"=w360:errorcluster, "Image Dst Out"=w361:T1)  [unwired: 8 in]
            n162 = call "Esophageal_CastImage.vi"("X Resolution"=w365, "Y Resolution"=w366, "error in (no error)"=w360, "Image In"=w361) -> ("error out"=w364:errorcluster)  [unwired: 7 in]
          }
        }
        n163 = local write "Recording"(FALSE ("Recording")) -> ()
        n164 = call-poly <vilib>:"DAQmx Read.vi"("task/channels in"=w143, "error in"=w130) -> ("task out"=w139:refnum<k21>, "data"=w142:bool[], "error out"=w134:errorcluster)  [unwired: 11 in]
        n165 = Index Array(array=w142, index=0) -> (element=w141:bool)
        n166 = Not(x=w141) -> (.not. x?=w140:bool)
        n167 = case shown="True" w140 {
          selector: w140 -> [w164 _]
          tunnel: w139 -> [w165 w179]
          tunnel: [w165 w178] -> w138
          tunnel: [w164 w177] -> w137
          tunnel: w134 -> [w163 w176]
          tunnel: [w163 w166] -> w129
          frame False {
          }
          frame True {
            w175 = T4."Disabled and Grayed Out" ("Disabled")
            # "Log Imaging Settings"
            # "Enable the pause button"
            # "Disable all controls on the front panel except the pause button"
            # "Waits until the foot pedal is done being pressed."
            n168 = while {
              tunnel: w179 -> [w187]
              tunnel: [w186] -> w178
              tunnel: [w182] -> w177
              tunnel: w176 -> [w183]
              tunnel: [w180] -> w173
              stop <- w181 stop-if-true
              n169 = call-poly <vilib>:"DAQmx Read.vi"("task/channels in"=w187, "error in"=w183) -> ("task out"=w186:refnum<k21>, "data"=w184:bool[], "error out"=w180:errorcluster)  [unwired: 11 in]
              n170 = Index Array(array=w184, index=0) -> (element=w182:bool)
              n171 = Or(x=w182, y=w180) -> (x .or. y?=w181:bool)
            }
            n172 = property on="Play Button" class="Bool"("DisabledEnum"=w175) -> ()  [unwired: 2 in, 2 out]
            n173 = property on="Calibrate" class="Bool"("DisabledEnum"=w175) -> ()  [unwired: 2 in, 2 out]
            n174 = property on="Close Program" class="Bool"("DisabledEnum"=w175) -> ()  [unwired: 2 in, 2 out]
            n175 = property on="Save Button" class="Bool"("DisabledEnum"=w175) -> ()  [unwired: 2 in, 2 out]
            n176 = property on="Pause Button" class="Bool"(error in=w173, "DisabledEnum"=T4."Enabled" ("Disabled")) -> (error out=w167:errorcluster)  [unwired: 1 in, 1 out]
            n177 = property on="HRME Exposure" class="Slide (strict)"("DisabledEnum"=w175) -> ()  [unwired: 2 in, 2 out]
            n178 = property on="HRME Gain" class="Slide (strict)"("DisabledEnum"=w175) -> ()  [unwired: 2 in, 2 out]
            n179 = local read "HRME Exposure"() -> (w171:dbl)
            n180 = local read "Auto Gain"() -> (w169:bool)
            n181 = property on="Auto Gain" class="Bool (strict)"("DisabledEnum"=w175) -> ()  [unwired: 2 in, 2 out]
            n182 = property on="Auto Exposure" class="Bool (strict)"("DisabledEnum"=w175) -> ()  [unwired: 2 in, 2 out]
            n183 = local read "Log File Out"() -> (w168:refnum<file>)
            n184 = local read "Auto Exposure"() -> (w170:bool)
            n185 = local read "HRME Gain"() -> (w172:dbl)
            n186 = call "Esophageal_Datalogger_PlayButton.vi"("Gain Value"=w172, "Auto Exposure Status"=w170, "error in (no error)"=w167, "Exposure Value"=w171, "Auto Gain Status"=w169, "Log File In"=w168) -> ("error out"=w166:errorcluster)  [unwired: 4 in, 1 out]
          }
        }
        n187 = Select(t=Esophogeal_Software_States."Imaging" ("Anal HRME States"), s=w137, f=w146) -> (s? t:f=w147:T2)
        n188 = Merge Errors(w133, w128, w129) -> (w132:errorcluster)
      }
      frame "Imaging" {
        # "Turn Red Light on to indicate frames are now being saved"
        n189 = while {
          tunnel: w405 -> [w451]
          tunnel: w404 -> [w450]
          tunnel: [w449] -> w403
          tunnel: [w428] -> w402
          tunnel: [w445] -> w390
          tunnel: w401 -> [w447]
          shift-right: [w442] -> w397
          shift-left: w400 -> [w448]
          tunnel: [w441] -> w396
          tunnel: [w439] -> w393
          tunnel: [w419] -> w389
          stop <- w440 stop-if-true
          w425 = T4."Disabled and Grayed Out" ("Disabled")
          w426 = T11 0 items=["Grayscale (U8)", "Grayscale (I16)", "Grayscale (SGL)", "Complex (CSG)", "RGB (U32)", "HSL (U32)", "RGB (U64)", "Grayscale (U16)"] ("Image Type")
          # "Converts image to array"
          # "Generate filename from timestamp"
          # "Send to producer"
          # "Read Foot Pedal Status"
          # "Acquire fastHRME Image"
          n190 = call <vilib>:"IMAQdx Grab2.vi"("error in"=w447, "Image In"=w450, "Session In"=w451) -> ("error out"=w427:errorcluster, "Image Out"=w428:T1, "Session Out"=w449:T8)  [unwired: 5 in, 1 out]
          n191 = call "IMAQ Cast Image 2"("Image Src"=w428, "Image Type"=w426, "error in (no error)"=w427) -> ("Image Dst Out"=w422:T1, "error out"=w421:errorcluster)  [unwired: 11 in]
          n192 = local write "HRME Image"(w422) -> ()
          n193 = local read "Height"() -> (w424:i16)
          n194 = local read "Width"() -> (w423:i16)
          n195 = Format Date/Time String(time format string (%c)="%H%M%S%3u") -> (date/time string=w431:string)  [unwired: 2 in]
          n196 = call "IMAQ ImageToArray"("Image"=w422) -> ("Image Pixels (U8)"=w432:u8[][])  [unwired: 3 in, 4 out]
          n197 = call-poly <vilib>:"DAQmx Read.vi"("task/channels in"=w448, "error in"=w447) -> ("task out"=w434:refnum<k21>, "data"=w436:bool[], "error out"=w433:errorcluster)  [unwired: 11 in]
          n198 = call "Esophageal_CastImage.vi"("X Resolution"=w423, "Y Resolution"=w424, "error in (no error)"=w421, "Image In"=w422) -> ("error out"=w420:errorcluster)  [unwired: 7 in]
          n199 = Concatenate Strings(w431, ".png" ("string")) -> (w419:string)
          n200 = call <extravilib>:"Write.vi"("element"=w419) -> ("channel"=w439:T13)  [unwired: 8 in, 2 out]
          n201 = Index Array(array=w436, index=0) -> (element=w437:bool)
          n202 = Not(x=w437) -> (.not. x?=w435:bool)
          n203 = case shown="True" w435 {
            selector: w435 -> [w453 _]
            tunnel: w434 -> [w454 w459]
            tunnel: [w454 w458] -> w442
            tunnel: [w453 w455] -> w443
            tunnel: w433 -> [w452 w457]
            tunnel: [w452 w456] -> w446
            frame False {
            }
            frame True {
              # "Waits until the foot pedal is done being pressed."
              n204 = while {
                tunnel: w459 -> [w466]
                tunnel: [w465] -> w458
                tunnel: [w462] -> w455
                tunnel: w457 -> [w461]
                tunnel: [w460] -> w456
                stop <- w462 stop-if-true
                n205 = call-poly <vilib>:"DAQmx Read.vi"("task/channels in"=w466, "error in"=w461) -> ("task out"=w465:refnum<k21>, "data"=w463:bool[], "error out"=w460:errorcluster)  [unwired: 11 in]
                n206 = Index Array(array=w463, index=0) -> (element=w462:bool)
              }
            }
          }
          n207 = property on="Save Button" class="Bool"("DisabledEnum"=w425) -> ()  [unwired: 2 in, 2 out]
          n208 = property on="Play Button" class="Bool"("DisabledEnum"=w425) -> ()  [unwired: 2 in, 2 out]
          n209 = property on="Image Analysis Meter" class="Slide (strict)"("DisabledEnum"=w425) -> ()  [unwired: 2 in, 2 out]
          n210 = Or(x="Pause Button", y=w443) -> (x .or. y?=w440:bool)
          "Pause Status" <- w440
          n211 = call <extravilib>:"Write.vi"("last element? (F)"=w440, "element"=w432) -> ("channel"=w441:T14)  [unwired: 7 in, 2 out]
          n212 = Merge Errors(w420, w446) -> (w445:errorcluster)
        }
        "Timestamp" <- w389
        n213 = call "IMAQ Create"("Image Name"="HRME Consumer") -> ("New Image"=w394:T1)  [unwired: 4 in, 1 out]
        n214 = while {
          tunnel: w396 -> [w418]
          shift-right: [w414] -> _
          shift-left: w394 -> [w410]
          tunnel: w393 -> [w413]
          stop <- w417 stop-if-true
          # "Reads image from channel, converts it into an image, then writes that image to file."
          n215 = local read "HRME Path"() -> (w409:path)
          n216 = call <extravilib>:"Read.vi"("channel"=w418) -> ("done?"=w417:bool, "element"=w416:u8[][])  [unwired: 6 in, 3 out]
          n217 = call <extravilib>:"Read.vi"("channel"=w413) -> ("element"=w411:string)  [unwired: 6 in, 4 out]
          n218 = call "IMAQ ArrayToImage"("Image Pixels (U8)"=w416, "Image"=w410) -> ("Image Out"=w415:T1)  [unwired: 8 in, 1 out]
          n219 = Build Path(base path=w409, name or relative path=w411) -> (appended path=w412:path)
          n220 = call-poly "IMAQ Write File 2"("Image Quality"=u32 1000, "File Path"=w412, "Image"=w415) -> ("Image Out (duplicate)"=w414:T1)  [unwired: 7 in, 1 out]
        }
        n221 = local read "Log File Out"() -> (w391:refnum<file>)
        n222 = call "Esophageal_Datalogger_PauseButton.vi"("error in (no error)"=w390, "Log File In"=w391) -> ("error out"=w392:errorcluster)  [unwired: 8 in, 1 out]
        "Recording" <- TRUE ("Recording")
      }
      frame "Exit" {
        # "Tell the python program to close"
        n223 = local read "Command File Location"() -> (w473:path)
        n224 = Bundle By Name(cluster=T6 {"Source"="", "Destination"="", "CMD"="newfolders", "Time"="time"} ("Output JSON File"), "CMD"="stop") -> (w476:T6)
        n225 = Flatten To JSON(anything=w476, error in (no error)=w471) -> (JSON string=w475:string, 11:w474:errorcluster)  [unwired: 1 in]
        n226 = Write to Text File(file (use dialog)=w473, text=w475, error in=w474) -> (error out=w470:errorcluster)  [unwired: 1 in, 2 out]
        n227 = local read "Log File Out"() -> (w469:refnum<file>)
        n228 = call "Esophageal_Datalogger_EndButton.vi"("error in (no error)"=w470, "Log File In"=w469) -> ("error out"=w468:errorcluster)  [unwired: 8 in, 1 out]
      }
    }
    "Software States" <- w26
    "error out" <- w17
  }
  n229 = property on="Play Button" class="Bool"("DisabledEnum"=w5) -> ()  [unwired: 2 in, 2 out]
  n230 = property on="HRME Exposure" class="Slide (strict)"("DisabledEnum"=w5) -> ()  [unwired: 2 in, 2 out]
  n231 = property on="Calibrate" class="Bool"("DisabledEnum"=w5) -> ()  [unwired: 2 in, 2 out]
  n232 = property on="HRME Gain" class="Slide (strict)"("DisabledEnum"=w5) -> ()  [unwired: 2 in, 2 out]
  n233 = property on="Close Program" class="Bool"("DisabledEnum"=w5) -> ()  [unwired: 2 in, 2 out]
  n234 = property on="Auto Gain" class="Bool (strict)"("DisabledEnum"=w5) -> ()  [unwired: 2 in, 2 out]
  n235 = property on="Save Button" class="Bool"("DisabledEnum"=w5) -> ()  [unwired: 2 in, 2 out]
  n236 = property on="Auto Exposure" class="Bool (strict)"("DisabledEnum"=w5) -> ()  [unwired: 2 in, 2 out]
  n237 = property on="Image Analysis Meter" class="Slide (strict)"("BG Color"=u32 0 ("Slider Colors:BG Color")) -> ()  [unwired: 2 in, 2 out]
  n238 = call <vilib>:"DAQmx Clear Task.vi"("task in"=w9, "error in"=w8) -> ("error out"=w1:errorcluster)  [unwired: 13 in]
  n239 = Close Python Session(session in=w2, error in=w1) -> ()  [unwired: 1 out]
